vi "OP300ZP_CONTI_VI.vi"(6 "Dernier Point en entrée":bool, 7 "OUI/NON":bool, 8 "entrée d'erreur (pas d'erreur)":errorcluster) -> (0 "sortie d'erreur":errorcluster, 1 "Dernier Point en sortie":bool, 2 "Compt":i32, 3 "Dernier Point 3":bool)   [LabVIEW 2020]
uses:
  <vilib>/Sylvain.lib/02 SLIM ZEN WS 500/SubVi/FGV.ctl
  VG/R.vi
panel:
  in  "cluster d'entrée":T1
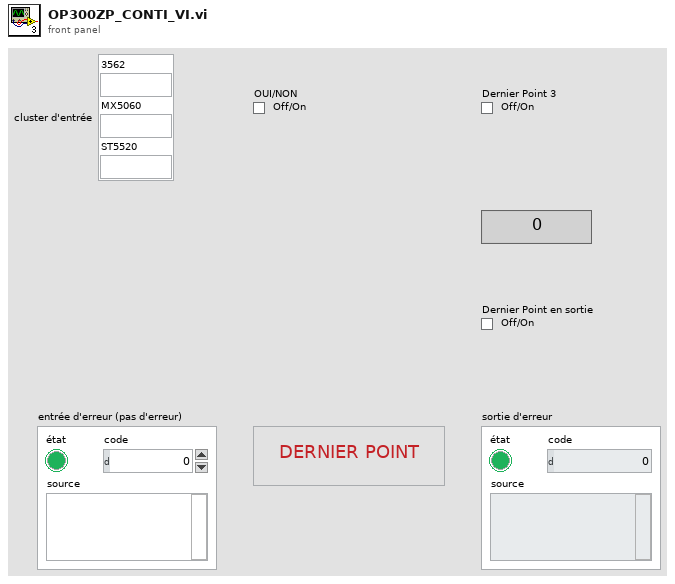
[diagram p1: front panel]
types:
  T1 = cluster{"3562":string, "MX5060":string, "ST5520":string}
  T2 = typedef "FGV.ctl" = enum16{"GET", "SET", "RAZ"}
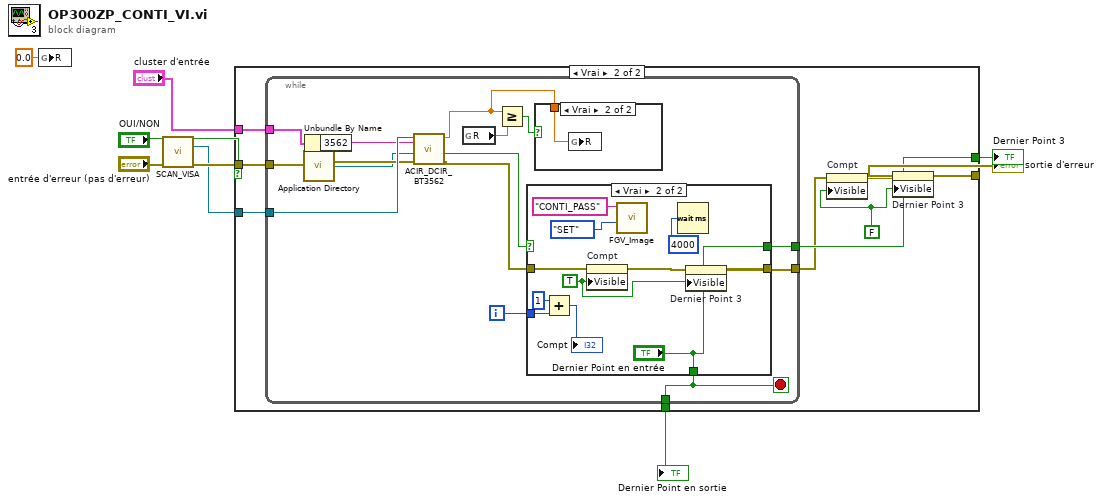
[diagram p0: block diagram]
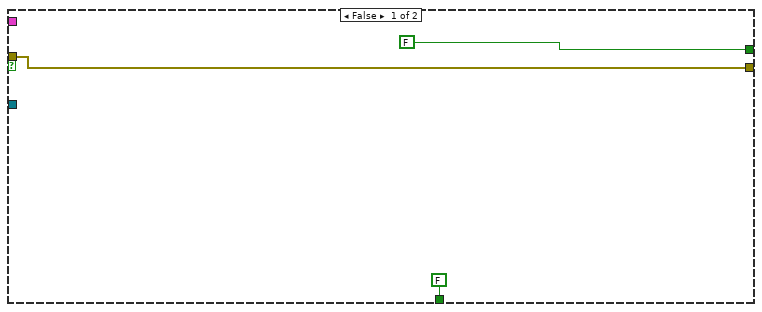
[diagram p2: hidden frame]
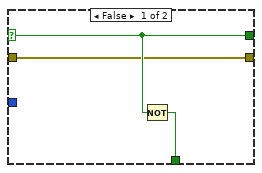
[diagram p3: hidden frame]
diagram:
  n1 = global write "R.vi" "R"(0.0 ("R")) -> ()
  n2 = call "SCAN_VISA.vi"("entrée d'erreur (pas d'erreur)"="entrée d'erreur (pas d'erreur)") -> ("sortie d'erreur"=w9:errorcluster, "Refnum VISA en sortie"=w2:refnum<visa-resource-name>)  [unwired: 9 in]
  n3 = case shown="Vrai" "OUI/NON" {
    tunnel: w2 -> [_ w21]
    tunnel: w9 -> [w12 w20]
    tunnel: [w12 w17] -> w5
    tunnel: [FALSE ("OUI/NON") w19] -> w6
    tunnel: [FALSE w18] -> w8
    tunnel: "cluster d'entrée" -> [_ w13]
    frame False {
    }
    frame True {
      w14 = FALSE ("Visible")
      n4 = while {
        tunnel: w21 -> [w35]
        tunnel: w20 -> [w34]
        tunnel: [w31] -> w16
        tunnel: [w26] -> w19
        tunnel: [w25] -> w18
        tunnel: w13 -> [w22]
        i -> [w30]
        stop <- w25 stop-if-true
        n5 = call <vilib>:"Application Directory.vi"() -> ("Application Directory"=w33:path)
        n6 = Unbundle By Name(w22) -> ("3562"=w23:string)
        n7 = call <userlib>:"ACIR_DCIR_BT3562.vi"("errin"=w34, "chemin de base"=w33, "section"=w23, "VISAin"=w35) -> ("errout"=w24:errorcluster, "R pass"=w32:bool, "R Out float"=w27:dbl)  [unwired: 5 out]
        n8 = global read "R.vi" "R"() -> (w29:dbl)
        n9 = Greater Or Equal?(x=w27, y=w29) -> (x >= y?=w28:bool)
        n10 = case shown="Vrai" w32 {
          selector: w32 -> [w38 _]
          tunnel: w24 -> [w36 w45]
          tunnel: [w36 w41] -> w31
          tunnel: [w37 "Dernier Point en entrée"] -> w25
          tunnel: w30 -> [_ w47]
          tunnel: [w38 "Dernier Point en entrée"] -> w26
          frame False {
            n11 = Not(x=w38) -> (.not. x?=w37:bool)
          }
          frame True {
            w39 = TRUE ("Visible")
            n12 = Add(x=1, y=w47) -> (x+y=→"Compt":i32)
            n13 = property on="Compt" class="NumNb (strict)"(error in=w45, "Visible"=w39) -> (error out=w42:errorcluster)  [unwired: 1 in, 1 out]
            n14 = call <vilib>:"FGV_Image.vi"("Énum"=FGV."SET", "IN"="CONTI_PASS") -> ()  [unwired: 9 in, 1 out]
            n15 = Wait (ms)(milliseconds to wait=u32 4000 ("attente (ms)")) -> ()  [unwired: 1 out]
            n16 = property on="Dernier Point 3" class="Bool (strict)"(error in=w42, "Visible"=w39) -> (error out=w41:errorcluster)  [unwired: 1 in, 1 out]
          }
        }
        n17 = case shown="Vrai" w28 {
          tunnel: w27 -> [_ w50]
          frame False {
          }
          frame True {
            n18 = global write "R.vi" "R"(w50) -> ()
          }
        }
      }
      n19 = property on="Compt" class="NumNb (strict)"(error in=w16, "Visible"=w14) -> (error out=w15:errorcluster)  [unwired: 1 in, 1 out]
      n20 = property on="Dernier Point 3" class="Bool (strict)"(error in=w15, "Visible"=w14) -> (error out=w17:errorcluster)  [unwired: 1 in, 1 out]
    }
  }
  "Dernier Point en sortie" <- w8
  "Dernier Point 3" <- w6
  "sortie d'erreur" <- w5
